vi "MotorPosReade.vi"() -> (0 "坐标输出":i32[](array[numeric]))   [LabVIEW 2018]
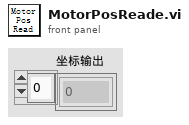
[diagram p1: front panel]
types:
  T1 = cluster{"激光器型号":string, "X":dbl, "Y":dbl, "Z":dbl, "Rotate":dbl, "Pitching":dbl}
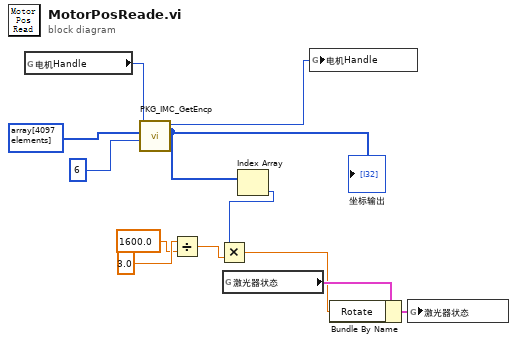
[diagram p0: block diagram]
diagram:
  n1 = global read "参数.vi" "电机Handle"() -> (w12:u32)
  n2 = call "PKG_IMC_GetEncp.vi"("axisnum"=6, "pos"=i32[] array[4097 elements], "Handle"=w12) -> ("pos out"=w6:i32[], "Handle out"=w11:u32)  [unwired: 6 in, 1 out]
  "坐标输出" <- w6
  n3 = Divide(x=3.0 ("y"), y=1600.0 ("x")) -> (x/y=w3:dbl)
  n4 = global read "参数.vi" "激光器状态"() -> (w8:T1)
  n5 = Index Array(array=w6) -> (element=w2:i32)  [unwired: 1 in]
  n6 = Multiply(x=w2, y=w3) -> (x*y=w1:dbl)
  n7 = global write "参数.vi" "电机Handle"(w11) -> ()
  n8 = Bundle By Name(cluster=w8, "Rotate"=w1) -> (w7:T1)
  n9 = global write "参数.vi" "激光器状态"(w7) -> ()
